vi "velocityPlanning.vi"(0 "Game in":refnum<class "Game.lvclass">, 1 "id":i32, 4 "robots":T2[](array[typedef]), 5 "error in (no error)":errorcluster, 6 "start":bool, 7 "V_sent":dbl=3.0 format="%#_13g", 9 "v_desired":dbl, 10 "v_sample":dbl, 11 "Dest":dbl[](array[numeric])=[4500.0, 3000.0] format="%#_13g", 12 "delta":dbl) -> (13 "velocityBreakState":T1, 14 "Game out":refnum<class "Game.lvclass">, 15 "TestTeam":refnum<class "Ally.lvclass">, 18 "replace":bool, 19 "error out":errorcluster)   [LabVIEW 2020, in "Game.lvclass"]
uses:
  Game.lvclass
  Communication_class/Paths/grSim Packet Command UDP Test Folder/grSim/grSim RobotReplacement.ctl
  Ally_class/Ally.lvclass
  C:/RoboIME/SSL_AI/Team_class/Team.lvclass
  Controls/velocityBreakState.ctl
  Game.lvclass/Game.ctl
  Team_class/Team.lvclass/Team.ctl
  Object_class/Object.lvclass/Object.ctl
  Object_class/Read x.vi
  Object_class/Read y.vi
  Read AllyRef.vi
  Team_class/Read RobotRef.vi
  Team_class/Write RobotRef.vi
  Robot_class/Robot.lvclass
  C:/RoboIME/SSL_AI/Object_class/Object.lvclass
  Utilities_class/Utilities.lvclass
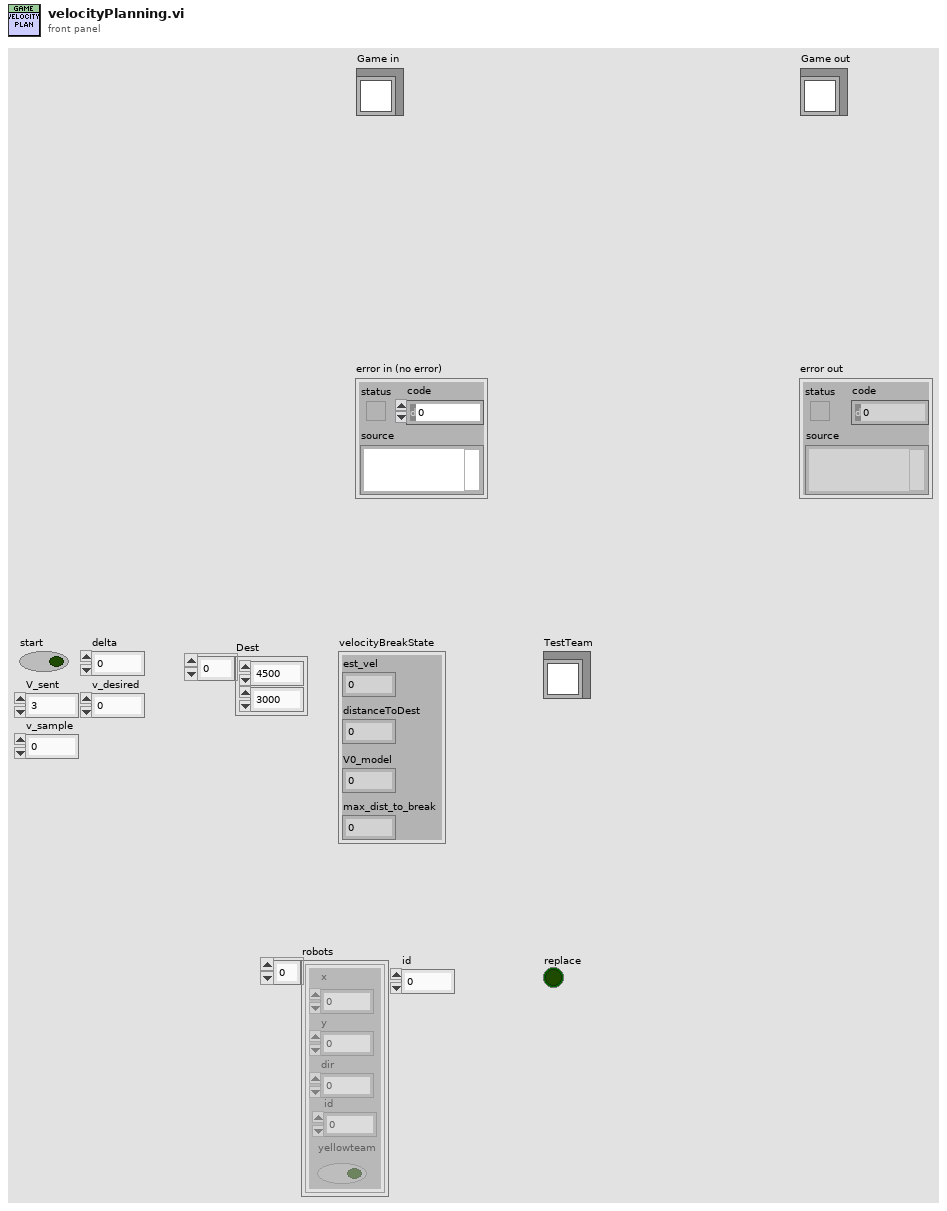
[diagram p1: front panel]
types:
  T1 = typedef "velocityBreakState.ctl" = cluster{"est_vel":dbl, "distanceToDest":dbl, "V0_model":dbl, "max_dist_to_break":dbl}
  T2 = typedef "grSim RobotReplacement.ctl" = cluster{"x":dbl, "y":dbl, "dir":dbl, "yellowteam":bool, "id":u32}
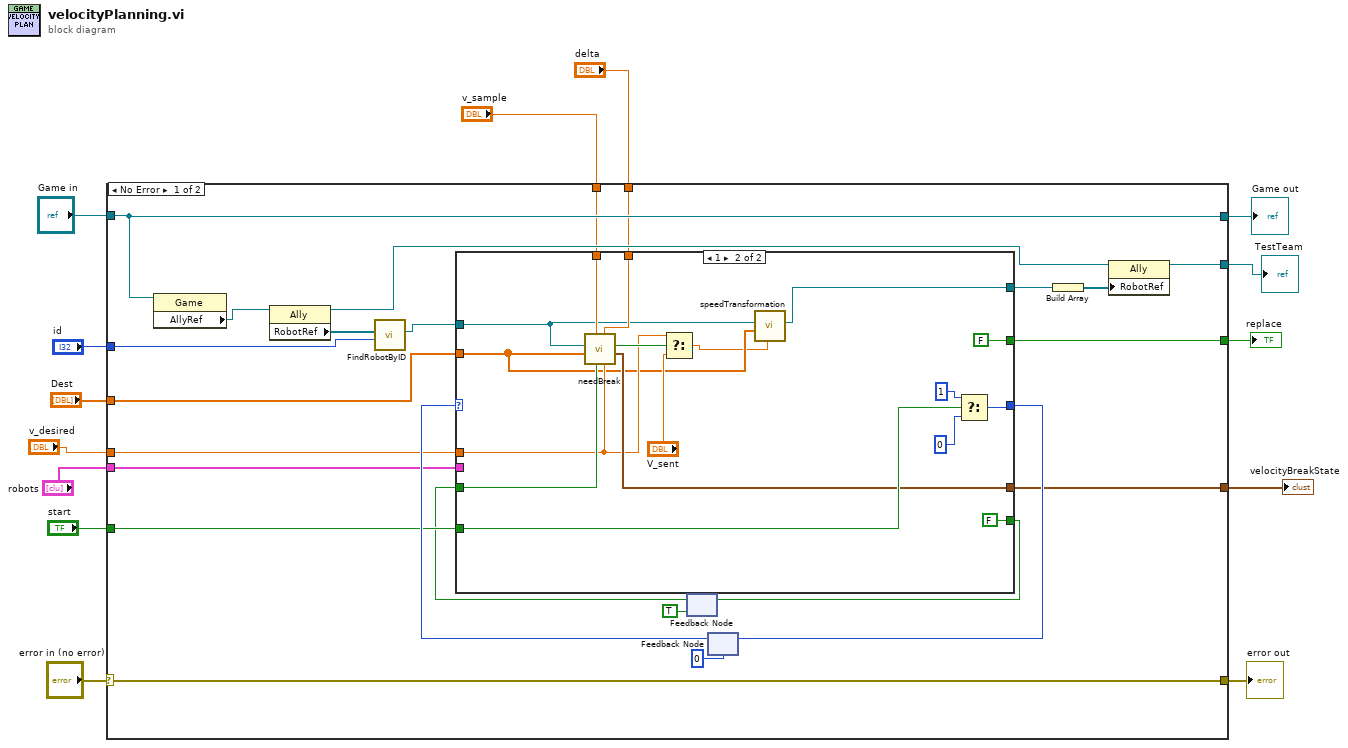
[diagram p0: block diagram]
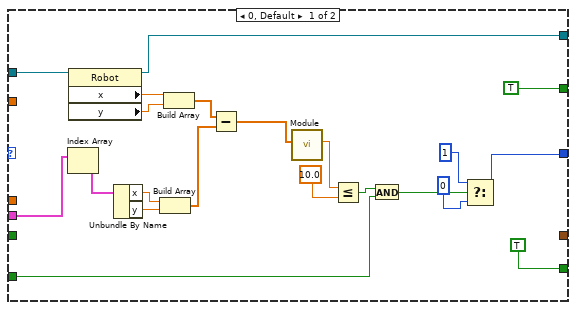
[diagram p2: hidden frame]
diagram:
  n1 = case shown="No Error" "error in (no error)" {
    selector: "error in (no error)" -> [w38 w78]
    tunnel: [w38 w78] -> w13
    tunnel: [w29 w77] -> w11
    tunnel: "Game in" -> [w29 w77]
    tunnel: "id" -> [w28 _]
    tunnel: "robots" -> [w27 _]
    tunnel: [w26 _] -> w8
    tunnel: [w24 _] -> w7
    tunnel: "Dest" -> [w23 _]
    tunnel: "start" -> [w22 _]
    tunnel: [w18 _] -> w4
    tunnel: "v_sample" -> [w17 _]
    tunnel: "delta" -> [w16 _]
    tunnel: "v_desired" -> [w15 _]
    frame No Error {
      n2 = property class="Game"(reference=w29) -> ("AllyRef"=w37:refnum<class "Ally.lvclass">)  [unwired: 1 in, 2 out]
      n3 = property class="Ally"(reference=w37) -> (reference out=w30:refnum<class "Ally.lvclass">, "RobotRef"=w36:refnum<class "Robot.lvclass">[])  [unwired: 1 in, 1 out]
      n4 = call "FindRobotByID.vi"("id"=w28, "RobotRef"=w36) -> ("Robot"=w34:refnum<class "Robot.lvclass">)  [unwired: 6 in, 3 out]
      n5 = feedback #1(TRUE) -> (w20:bool)
      n6 = feedback #2(0) -> (w35:i32)
      n7 = case shown="1" w35 {
        tunnel: w34 -> [w49 w63]
        tunnel: w27 -> [w48 _]
        tunnel: [TRUE FALSE] -> w26
        tunnel: [w44 w71] -> w33
        tunnel: [w43 w60] -> w32
        tunnel: w23 -> [_ w62]
        tunnel: w22 -> [w40 w74]
        tunnel: [TRUE FALSE] -> w21
        tunnel: w20 -> [_ w69]
        tunnel: [_ w68] -> w18
        tunnel: w17 -> [_ w67]
        tunnel: w16 -> [_ w66]
        tunnel: w15 -> [_ w65]
        frame 0, Default {
          n8 = Index Array(array=w48) -> (element=w56:T2)  [unwired: 1 in]
          n9 = property class="Robot"(reference=w49) -> (reference out=w43:refnum<class "Robot.lvclass">, "x"=w59:dbl, "y"=w58:dbl)  [unwired: 1 in, 1 out]
          n10 = Unbundle By Name(w56) -> ("x"=w55:dbl, "y"=w54:dbl)
          n11 = Build Array(w55, w54) -> (w53:dbl[])
          n12 = Build Array(w59, w58) -> (w57:dbl[])
          n13 = Subtract(x=w57, y=w53) -> (x-y=w52:dbl[])
          n14 = call "Module.vi"("2D vector"=w52) -> ("Modulo"=w51:dbl)  [unwired: 8 in, 2 out]
          n15 = Less Or Equal?(x=w51, y=10.0) -> (x <= y?=w41:bool)
          n16 = And(x=w41, y=w40) -> (x .and. y?=w42:bool)
          n17 = Select(t=1, s=w42, f=0) -> (s? t:f=w44:i32)
        }
        frame 1 {
          n18 = call "needBreak.vi"("desired_vel"=w65, "delta"=w66, "firstCall"=w69, "v_sample"=w67, "dest"=w62, "Robot"=w63) -> ("velocityBreakState"=w68:T1, "needBreak"=w75:bool)  [unwired: 2 in, 2 out]
          n19 = Select(t=w65, s=w75, f="V_sent") -> (s? t:f=w61:dbl)
          n20 = call "speedTransformation.vi"("V_sent"=w61, "Dest"=w62, "Robot"=w63) -> ("Robot out"=w60:refnum<class "Robot.lvclass">)  [unwired: 6 in, 2 out]
          n21 = Select(t=1, s=w74, f=0) -> (s? t:f=w71:i32)
        }
      }
      n22 = feedback-in #1(w21) -> ()
      n23 = feedback-in #2(w33) -> ()
      n24 = Build Array(w32) -> (w31:refnum<class "Robot.lvclass">[])
      n25 = property class="Ally"(reference=w30, "RobotRef"=w31) -> (reference out=w24:refnum<class "Ally.lvclass">)  [unwired: 1 in, 1 out]
    }
    frame Error {
    }
  }
  "error out" <- w13
  "Game out" <- w11
  "replace" <- w8
  "TestTeam" <- w7
  "velocityBreakState" <- w4
